vi "Robot Main.vi"() -> ()   [LabVIEW 2011]
doc: "This VI imlements the framework and scheduler for your robotics program. It should not be necessary to modify the framework. You are expected to add your code to the VIs called from Robot Main, the ones located in the Team Code within the project."
uses:
  <vilib>/Rock Robotics/WPI/DriverStation/WPI_DriverStationRobotMode.ctl
  Robot Global Data.vi
panel:
  in  "Finish":bool
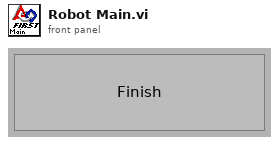
[diagram p1: front panel]
types:
  T1 = typedef "WPI_DriverStationRobotMode.ctl" = enum16{"Autonomous Disabled", "Autonomous Enabled", "Teleop Disabled", "Teleop Enabled", "Timeout", "Finish"}
  T2 = typedef "WPI_DriverStationMatch Info.ctl" = cluster{"Autonomous Elapsed Seconds":dbl, "TeleOp Elapsed Seconds":dbl, "Disabled Elapsed Seconds":dbl, "Visited Autonomous":bool, "Visited TeleOp":bool, "Visited Disabled":bool, "Autonomous Settings":cluster{"Autonomous Style":enum16{"Iterative", "Independent"}, "VI Refnum":refnum<vi>}}
  T3 = typedef "WPI_DriverStationDerivedRobotMode.ctl" = enum16{"Init", "Execute", "Stop"}
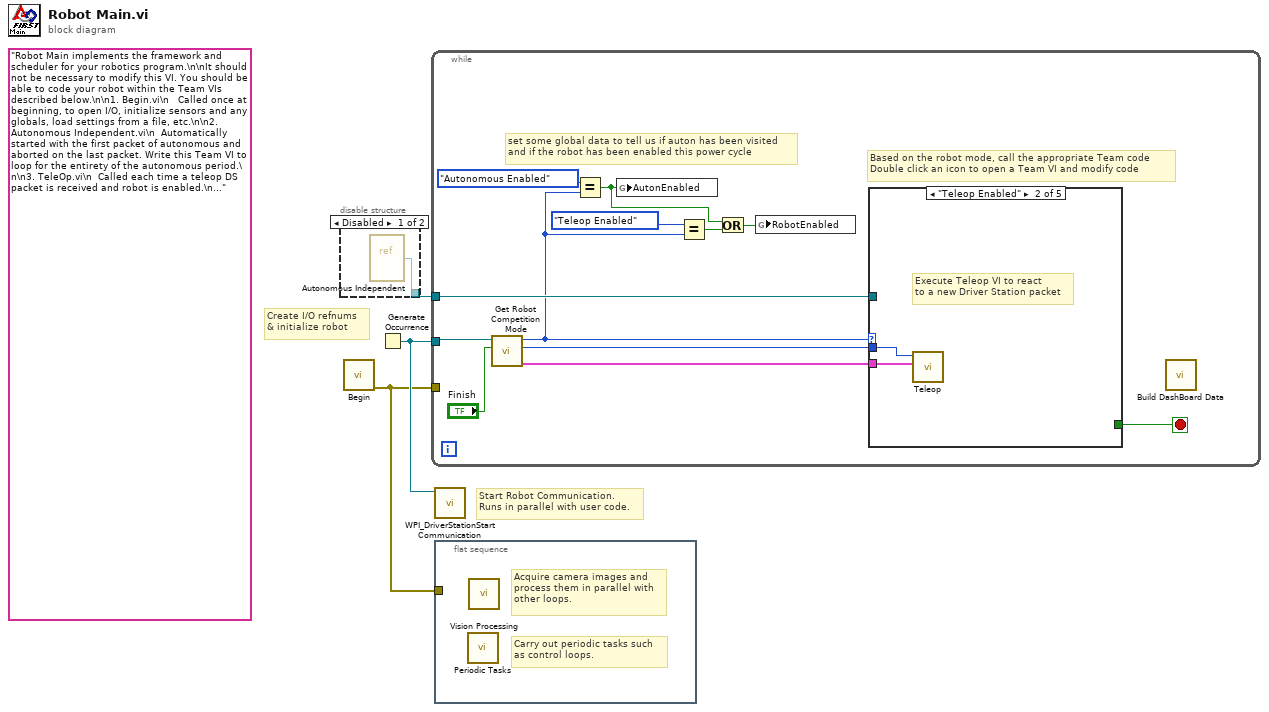
[diagram p0: block diagram]
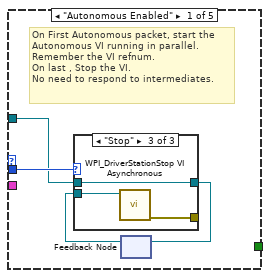
[diagram p3: hidden frame]
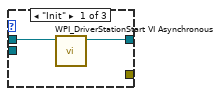
[diagram p4: hidden frame]
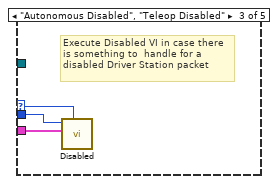
[diagram p6: hidden frame]
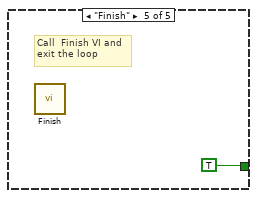
[diagram p8: hidden frame]
diagram:
  (unwired) "Robot Main implements the framework and scheduler for your robotics program.\n\nIt should not be necessary to modify this VI. You should be able to code your robot within the Team VIs described below.\n\n1. Begin.vi\n   Called once at beginning, to open I/O, initialize sensors and any globals, load settings from a file, etc.\n\n2. Autonomous Independent.vi\n  Automatically started with the first packet of autonomous and aborted on the last packet. Write this Team VI to loop for the entirety of the autonomous period.\n\n3. TeleOp.vi\n  Called each time a teleop DS packet is received and robot is enabled.\n\n4. Disabled.vi\n  Called each time a packet is received and the robot is disabled.\n\n5. Vision.vi\n  A parallel loop that acquires and processes camera images.\n\n6. PeriodicTasks.vi\n  Parallel loops running at user-defined rates.\n\n7. Finish.vi\n  Called before exiting, so you can save data, clean up I/O, etc.\n\n8. Build DashBoard Data.vi\n  Called for each driver station packet including timeouts. It is used to send select I/O values back to the Dashboard."
  # "Create I/O refnums\n& initialize robot"
  # "Start Robot Communication.\nRuns in parallel with user code."
  n1 = disable-structure shown="Disabled" {
    disable-tunnel: [w4 _] -> w1
    frame Disabled {
      n2 = vi-ref "Autonomous Independent.vi"() -> (w4:refnum<vi>)
    }
    frame Enabled {
    }
  }
  n3 = call "Begin.vi"() -> ("error out"=w2:errorcluster)  [unwired: 1 in, 10 out]
  n4 = Generate Occurrence() -> (w3:refnum<k4>)
  n5 = while {
    tunnel: w3 -> [w15]
    tunnel: w2 -> [_]
    tunnel: w1 -> [w11]
    stop <- w12 stop-if-true
    # "set some global data to tell us if auton has been visited\nand if the robot has been enabled this power cycle"
    # "Based on the robot mode, call the appropriate Team code\nDouble click an icon to open a Team VI and modify code"
    n6 = call "Get Robot Competition Mode.vi"("Finish"="Finish", "DS Occurrence"=w15) -> ("Match Info out"=w13:T2, "Call Context"=w16:T3, "Robot Mode"=w8:T1)  [unwired: 7 out]
    n7 = Equal?(x=WPI_DriverStationRobotMode."Autonomous Enabled", y=w8) -> (x = y?=w6:bool)
    n8 = global write "Robot Global Data.vi" "AutonEnabled"(w6) -> ()
    n9 = Equal?(x=WPI_DriverStationRobotMode."Teleop Enabled", y=w8) -> (x = y?=w7:bool)
    n10 = Or(x=w6, y=w7) -> (x .or. y?=w5:bool)
    n11 = global write "Robot Global Data.vi" "RobotEnabled"(w5) -> ()
    n12 = case shown="\"Teleop Enabled\"" w8 {
      selector: w8 -> [_ _ w29 _ _]
      tunnel: w16 -> [w20 w28 w31 _ _]
      tunnel: w13 -> [_ w27 w30 _ _]
      tunnel: [_ _ _ _ TRUE] -> w12
      tunnel: w11 -> [w19 _ _ _ _]
      frame "Autonomous Enabled" {
        # "On First Autonomous packet, start the\nAutonomous VI running in parallel.\nRemember the VI refnum.\nOn last , Stop the VI.\nNo need to respond to intermediates."
        n13 = feedback #1() -> (w17:refnum<vi>)  [unwired: 1 out]
        n14 = case shown="\"Stop\"" w20 {
          tunnel: w19 -> [w22 _ w25]
          tunnel: [w21 w23 w25] -> w18
          tunnel: w17 -> [_ w23 w26]
          tunnel: [_ _ w24] -> _
          frame "Init" {
            n15 = call <vilib>:"WPI_DriverStationStart VI Asynchronous.vi"("VI"=w22) -> ("VI out"=w21:refnum<vi>)  [unwired: 10 out]
          }
          frame "Execute", Default {
            # "Nothing to do"
          }
          frame "Stop" {
            n16 = call <vilib>:"WPI_DriverStationStop VI Asynchronous.vi"("VI Refnum"=w26) -> ("error out"=w24:errorcluster)  [unwired: 10 out]
          }
        }
        n17 = feedback-in #1(w18) -> ()
      }
      frame "Teleop Enabled" {
        # "Execute Teleop VI to react\nto a new Driver Station packet"
        n18 = call "Teleop.vi"("Match Info"=w27, "Call Context"=w28) -> ()  [unwired: 1 in, 9 out]
      }
      frame "Autonomous Disabled", "Teleop Disabled" {
        # "Execute Disabled VI in case there\nis something to  handle for a\ndisabled Driver Station packet"
        n19 = call "Disabled.vi"("Robot Mode"=w29, "Match Info"=w30, "Call Context"=w31) -> ()  [unwired: 1 in, 8 out]
      }
      frame "Timeout" {
        # "Driver Station packet didn't arrive.\nPossibly useful for diagnostics"
      }
      frame "Finish" {
        # "Call  Finish VI and\nexit the loop"
        n20 = call "Finish.vi"() -> ()  [unwired: 1 in, 7 out]
      }
    }
    n21 = call "Build DashBoard Data.vi"() -> ()  [unwired: 1 in, 11 out]
  }
  n22 = call <vilib>:"WPI_DriverStationStart Communication.vi"("occurrence"=w3) -> ()  [unwired: 11 out]
  n23 = flat-sequence {
    tunnel: w2 -> [_]
    frame #0 {
      # "Carry out periodic tasks such\nas control loops."
      # "Acquire camera images and\nprocess them in parallel with\nother loops."
      n24 = call "Periodic Tasks.vi"() -> ()  [unwired: 1 in, 11 out]
      n25 = call "Vision Processing.vi"() -> ()  [unwired: 1 in, 7 out]
    }
  }
